vi "CalCheckRatios.vi"() -> (5 "Plug in titles":string[](array[string]), 7 "Plug in values":string[](array[string]))   [LabVIEW 2011]
uses:
  Globals/Meas_global.vi
panel:
  out "Status":bool[](array[boolean])
  in  "Tolerance":dbl=3.0 format="%.1g%%"
  out "Value":dbl format="%.2g"
  out "Error":dbl[](array[numeric]) format="%.1g%%"
  out "Values":dbl[](array[numeric]) format="%.2g"
  in  "CalCheckChannels":u16[](array[ring]) items=["Inst name", "Pitot (Ucal)", "HW (HF1)", "HW (HF2)", "HW (HF3)", "Gen (1101)", "Gen (1102)", "Gen (1103)", "Gen (1104)", "Gen (1105)", "Gen (1106)", "Gen (1107)", "Gen (1108)", "Gen (1201)", "Gen (1202)", "Gen (1203)", "Gen (1204)", "Gen (1205)", "Gen (1206)", "Gen (1301)", "Gen (1302)", "Gen (1303)", "Gen (1304)", "Gen (1305)", "Gen (1306)", "Gen (1307)", "Gen (1308)", "Gen (2101)", "Gen (2102)", "Gen (2103)", "Gen (2104)", "Gen (2201)", "Gen (2202)", "Gen (2203)", "Gen (2204)", "Gen (2301)", "Gen (2302)", "Gen (2303)", "Gen (2304)", "Gen (2401)", "Gen (2402)", "Gen (2403)", "Gen (2404)", "Gen (3101)", "Gen (3201)", "Gen (3202)", "Gen (3301)", "Gen (3302)", "Gen (3401)", "Gen (3402)", "Gen (3501)", "Gen (3502)", "Gen (3601)", "Gen (3602)", "Gen (3701)", "Gen (3702)", "Gen (3801)", "Gen (3802)", "Gen (3901)", "Gen (3902)", "Gen (3903)", "Gen (4101)", "Gen (4102)", "Gen (4103)", "Gen (4104)", "Gen (4105)", "Gen (4106)", "Gen (Quiet)", "Gen (Pref)"]
  in  "Reference":u16(ring) items=["Inst name", "Pitot (Ucal)", "HW (HF1)", "HW (HF2)", "HW (HF3)", "Gen (1101)", "Gen (1102)", "Gen (1103)", "Gen (1104)", "Gen (1105)", "Gen (1106)", "Gen (1107)", "Gen (1108)", "Gen (1201)", "Gen (1202)", "Gen (1203)", "Gen (1204)", "Gen (1205)", "Gen (1206)", "Gen (1301)", "Gen (1302)", "Gen (1303)", "Gen (1304)", "Gen (1305)", "Gen (1306)", "Gen (1307)", "Gen (1308)", "Gen (2101)", "Gen (2102)", "Gen (2103)", "Gen (2104)", "Gen (2201)", "Gen (2202)", "Gen (2203)", "Gen (2204)", "Gen (2301)", "Gen (2302)", "Gen (2303)", "Gen (2304)", "Gen (2401)", "Gen (2402)", "Gen (2403)", "Gen (2404)", "Gen (3101)", "Gen (3201)", "Gen (3202)", "Gen (3301)", "Gen (3302)", "Gen (3401)", "Gen (3402)", "Gen (3501)", "Gen (3502)", "Gen (3601)", "Gen (3602)", "Gen (3701)", "Gen (3702)", "Gen (3801)", "Gen (3802)", "Gen (3901)", "Gen (3902)", "Gen (3903)", "Gen (4101)", "Gen (4102)", "Gen (4103)", "Gen (4104)", "Gen (4105)", "Gen (4106)", "Gen (Quiet)", "Gen (Pref)"]
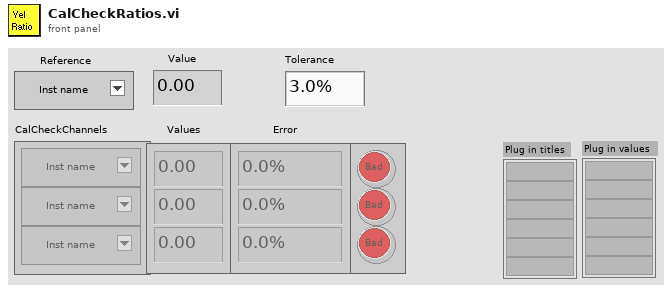
[diagram p1: front panel]
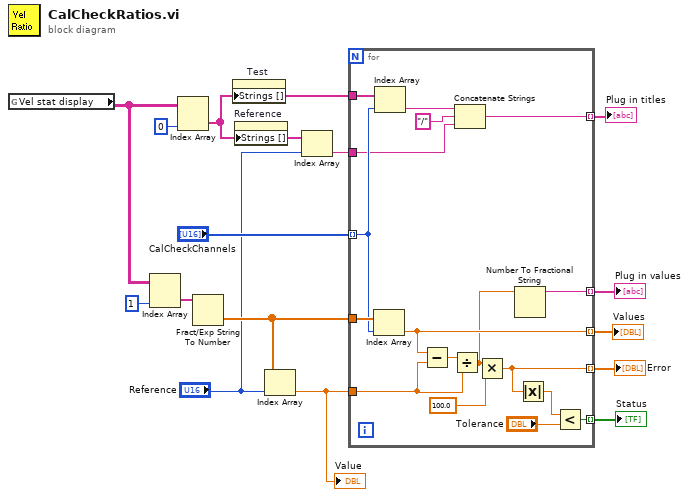
[diagram p0: block diagram]
diagram:
  n1 = global read "Meas_global.vi" "Vel stat display"() -> (w15:string[][])
  n2 = Index Array(array=w15, index (col)=1 ("index")) -> (element=w12:string[])  [unwired: 1 in]
  n3 = Index Array(array=w15, index (col)=0 ("index")) -> (element=w5:string[])  [unwired: 1 in]
  n4 = Fract/Exp String To Number(string=w12) -> (number=w10:dbl[])  [unwired: 3 in, 1 out]
  n5 = property on="Test" class="Ring (strict)"("Strings []"=w5) -> ()  [unwired: 2 in, 2 out]
  n6 = property on="Reference" class="Ring (strict)"("Strings []"=w5) -> ()  [unwired: 2 in, 2 out]
  n7 = Index Array(array=w10, index="Reference") -> (element=w7:dbl)
  "Value" <- w7
  n8 = Index Array(array=w5, index="Reference") -> (element=w3:string)
  n9 = for {
    tunnel: w10 -> [w32]
    tunnel: "CalCheckChannels" -> [w22] mode=indexing
    tunnel: [w31] -> w9 mode=indexing
    tunnel: w7 -> [w29]
    tunnel: [w27] -> w8 mode=indexing
    tunnel: [w25] -> w6 mode=indexing
    tunnel: w5 -> [w23]
    tunnel: w3 -> [w20]
    tunnel: [w18] -> w2 mode=indexing
    tunnel: [w16] -> w1 mode=indexing
    n10 = Index Array(array=w32, index=w22) -> (element=w31:dbl)
    n11 = Index Array(array=w23, index=w22) -> (element=w21:string)
    n12 = Subtract(x=w31, y=w29) -> (x-y=w30:dbl)
    n13 = Divide(x=w30, y=w29) -> (x/y=w17:dbl)
    n14 = Concatenate Strings(w21, "/" ("string"), w20) -> (w18:string)
    n15 = Multiply(x=w17, y=100.0) -> (x*y=w27:dbl)
    n16 = Number To Fractional String(number=w17) -> (F-format string=w16:string)  [unwired: 3 in]
    n17 = Absolute Value(x=w27) -> (abs(x)=w24:dbl)
    n18 = Less?(x=w24, y="Tolerance") -> (x < y?=w25:bool)
  }
  "Plug in values" <- w1
  "Plug in titles" <- w2
  "Values" <- w9
  "Error" <- w8
  "Status" <- w6
